vi "8digitDisplay7segment.vi"   [LabVIEW 2014]
uses:
  QwaveSys_Interface/QwaveSys_Interface.lvlib
  <vilib>/Aledyne-TSXperts/Arduino Compatible Compiler for LabVIEW/Arduino Compatible Compiler for LabVIEW.lvlib
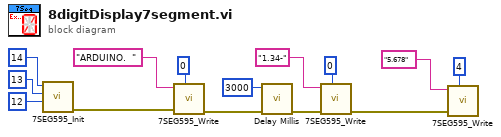
[diagram p0: block diagram]
diagram:
  n1 = call "7SEG595_Init.vi"("DIO"=u8 12, "RCLK"=u8 13, "SCLK"=u8 14) -> ("error out"=w8:errorcluster)  [unwired: 8 in]
  n2 = call "7SEG595_Write.vi"("index"=u8 0, "error in (no error)"=w8, "data"="ARDUINO.  ") -> ("error out"=w2:errorcluster)  [unwired: 8 in]
  n3 = call <vilib>:"Delay Millis.vi"("error in (no error)"=w2, "delay"=u32 3000) -> ("error out"=w3:errorcluster)  [unwired: 9 in]
  n4 = call "7SEG595_Write.vi"("index"=u8 0, "error in (no error)"=w3, "data"="1.34-") -> ("error out"=w10:errorcluster)  [unwired: 8 in]
  n5 = call "7SEG595_Write.vi"("index"=u8 4, "error in (no error)"=w10, "data"="5.678") -> ()  [unwired: 8 in, 1 out]
